vi "Ctor.vi"(7 "Mode (Raw)":T1, 8 "error in (no error)":errorcluster, 11 "Connection in":refnum<class "Connection.lvclass">) -> (0 "error out":errorcluster, 3 "Connection out":refnum<class "Connection.lvclass">)   [LabVIEW 2020, in "Stream.lvlib" / "Connection.lvclass"]
uses:
  Connection.lvclass
  Mode.ctl
  Ref Data.ctl
  State.ctl
  Connection.lvclass/Connection.ctl
  Endpoint/Endpoint.lvclass
  Stream.lvlib
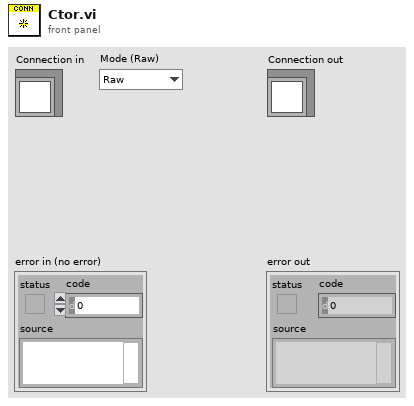
[diagram p1: front panel]
types:
  T1 = typedef "Stream.lvlib/Mode.ctl" = enum16{"Raw", "Buffered", "LineTerm", "Message"}
  T2 = typedef "Stream.lvlib/Connection.lvclass/Ref Data.ctl" = cluster{"State":T3}
  T3 = typedef "Stream.lvlib/Connection.lvclass/State.ctl" = enum16{"Closed", "Idle", "Connecting", "Connected", "Shutdown"}
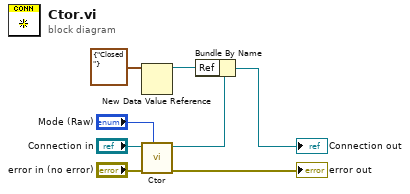
[diagram p0: block diagram]
diagram:
  n1 = New Data Value Reference(data value=T2 {"State"=enum."Closed"} ("Ref Data")) -> (data value reference=w3:refnum<data-value>)  [unwired: 1 in, 1 out]
  n2 = call-parent "Ctor.vi"("Mode (Raw)"="Mode (Raw)", "error in (no error)"="error in (no error)", "Endpoint in"="Connection in") -> ("error out"=→"error out":errorcluster, "Endpoint out"=w4:refnum<class "Connection.lvclass">)  [unwired: 7 in]
  n3 = Bundle By Name(cluster=w4, "Ref"=w3) -> (→"Connection out":refnum<class "Connection.lvclass">)
